vi "HEWH Determine Intellifaucet Setting.vi"(8 "Error In":errorcluster, 11 "GPM Target":dbl) -> (0 "Error Out":errorcluster, 3 "Valve % Open":dbl)   [LabVIEW 2016]
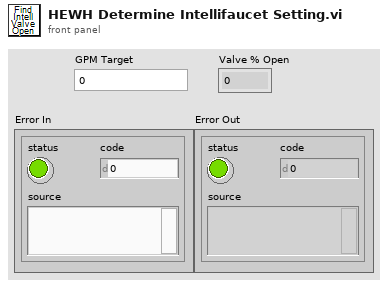
[diagram p1: front panel]
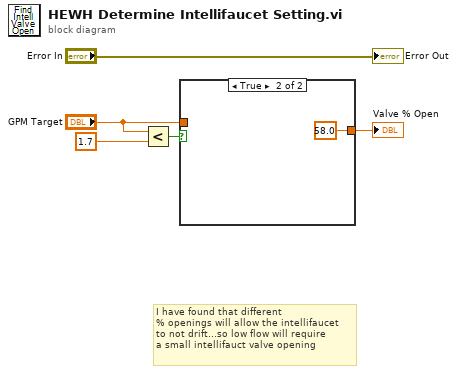
[diagram p0: block diagram]
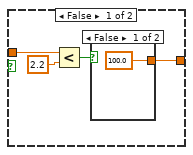
[diagram p2: hidden frame]
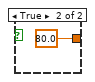
[diagram p3: hidden frame]
diagram:
  # "I have found that different\n% openings will allow the intellifaucet\nto not drift...so low flow will require\na small intellifauct valve opening"
  n1 = Less?(x="GPM Target", y=1.7) -> (x < y?=w4:bool)
  n2 = case shown="True" w4 {
    tunnel: [w6 58.0 ("Flow Rate (GPM)")] -> w2
    tunnel: "GPM Target" -> [w9 _]
    frame False {
      n3 = Less?(x=w9, y=2.2) -> (x < y?=w7:bool)
      n4 = case shown="False" w7 {
        tunnel: [100.0 ("Flow Rate (GPM)") 80.0 ("Flow Rate (GPM)")] -> w6
        frame False {
        }
        frame True {
        }
      }
    }
    frame True {
    }
  }
  "Valve % Open" <- w2
  "Error Out" <- "Error In"
